vi "Can Init.vi"   [LabVIEW 2023]
uses:
  <vilib>/xnet/xnet.llb/XNET Create Session (Frame Output Stream).vi
  <resource>/objmgr/xnet.rc
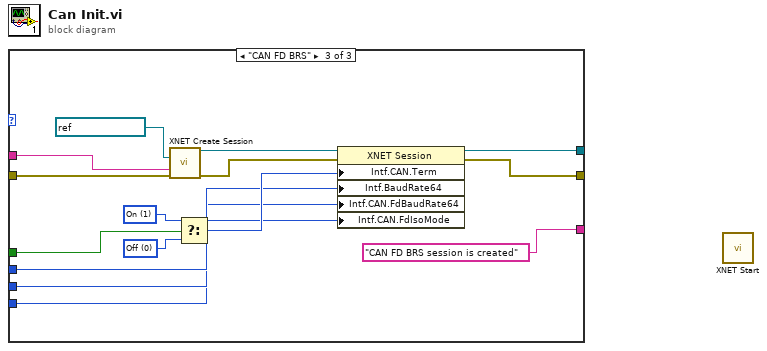
[diagram p0: block diagram]
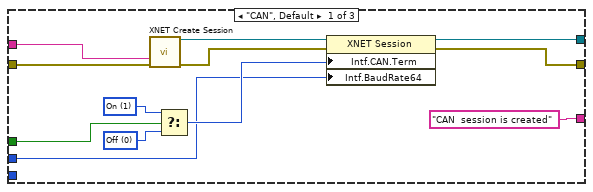
[diagram p2: hidden frame]
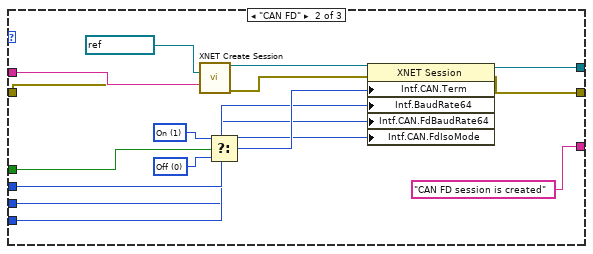
[diagram p3: hidden frame]
diagram:
  n1 = case shown="\"CAN FD BRS\"" {
    selector: _ -> [_ _ _]
    tunnel: [w7 w16 w36] -> _
    tunnel: _ -> [w2 w21 w31]
    tunnel: _ -> [w6 w20 w30]
    tunnel: [w5 w15 w29] -> _
    tunnel: _ -> [w4 w19 w35]
    tunnel: _ -> [w3 w18 w34]
    tunnel: _ -> [_ w14 w33]
    tunnel: _ -> [_ w17 w32]
    tunnel: ["CAN  session is created" ("message") "CAN FD session is created" ("message") "CAN FD BRS session is created" ("message")] -> _
    frame "CAN", Default {
      w10 = u32 1 items=["Off", "On"] ("Interface:CAN:Termination")
      w9 = u32 0 items=["Off", "On"] ("Interface:CAN:Termination")
      n2 = call-poly <vilib>:"XNET Create Session.vi"("interface"=w2, "error in (no error)"=w6) -> ("session out"=w12:refnum<k21>, "error out"=w11:errorcluster)  [unwired: 12 in]
      n3 = Select(t=w10, s=w4, f=w9) -> (s? t:f=w8:u32)
      n4 = property class="XNET Session"(reference=w12, error in=w11, "Intf.CAN.Term"=w8, "Intf.BaudRate64"=w3) -> (reference out=w7:refnum<k21>, error out=w5:errorcluster)
    }
    frame "CAN FD" {
      w24 = u32 1 items=["Off", "On"] ("Interface:CAN:Termination")
      w23 = u32 0 items=["Off", "On"] ("Interface:CAN:Termination")
      n5 = call-poly <vilib>:"XNET Create Session.vi"("cluster (:memory:)"=refnum<k21> ":can_fd:", "interface"=w21, "error in (no error)"=w20) -> ("session out"=w26:refnum<k21>, "error out"=w25:errorcluster)  [unwired: 11 in]
      n6 = Select(t=w24, s=w19, f=w23) -> (s? t:f=w22:u32)
      n7 = property class="XNET Session"(reference=w26, error in=w25, "Intf.CAN.Term"=w22, "Intf.BaudRate64"=w18, "Intf.CAN.FdBaudRate64"=w14, "Intf.CAN.FdIsoMode"=w17) -> (reference out=w16:refnum<k21>, error out=w15:errorcluster)
    }
    frame "CAN FD BRS" {
      w39 = u32 1 items=["Off", "On"] ("Interface:CAN:Termination")
      w38 = u32 0 items=["Off", "On"] ("Interface:CAN:Termination")
      n8 = call-poly <vilib>:"XNET Create Session.vi"("cluster (:memory:)"=refnum<k21> ":can_fd_brs:", "interface"=w31, "error in (no error)"=w30) -> ("session out"=w41:refnum<k21>, "error out"=w40:errorcluster)  [unwired: 11 in]
      n9 = Select(t=w39, s=w35, f=w38) -> (s? t:f=w37:u32)
      n10 = property class="XNET Session"(reference=w41, error in=w40, "Intf.CAN.Term"=w37, "Intf.BaudRate64"=w34, "Intf.CAN.FdBaudRate64"=w33, "Intf.CAN.FdIsoMode"=w32) -> (reference out=w36:refnum<k21>, error out=w29:errorcluster)
    }
  }
  n11 = call <vilib>:"XNET Start.vi"() -> ()  [unwired: 14 in, 2 out]
